vi "HSE Logger - Log Handlers and Levels.vi"(8 "error in":errorcluster) -> (0 "error out":errorcluster)   [LabVIEW 2024]
uses:
  <vilib>/Utility/error.llb/Trim Whitespace One-Sided.vi
  <vilib>/Hampel Software Engineering/HSE Logger/Handler/Handler.lvclass
  <vilib>/Hampel Software Engineering/HSE Logger/hse-logger.lvlib
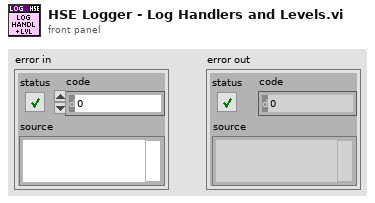
[diagram p1: front panel]
types:
  T1 = typedef "hse-logger.lvlib/LogLevel.ctl" = enum16{"DEBUG", "INFO", "WARNING", "ERROR", "CRITICAL"}
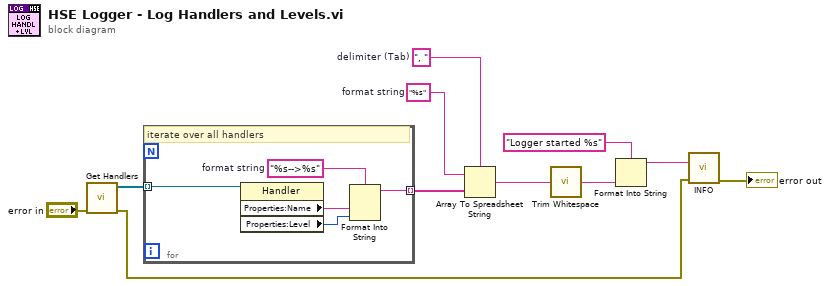
[diagram p0: block diagram]
diagram:
  w5 = ", "  # delimiter (Tab)
  w6 = "%s"  # format string
  n1 = call <vilib>:"Get Handlers.vi"("error in"="error in") -> ("error out"=w10:errorcluster, "Handlers"=w8:refnum<class "Handler.lvclass">[])  [unwired: 9 in]
  n2 = for {
    tunnel: w8 -> [w16] mode=indexing
    tunnel: [w12] -> w7 mode=indexing
    w15 = "%s-->%s"  # format string
    # "iterate over all handlers"
    n3 = property class="Handler"(reference=w16) -> ("Properties:Name"=w14:string, "Properties:Level"=w13:T1)  [unwired: 1 in, 2 out]
    n4 = Format Into String(format string=w15, w14, w13) -> (resulting string=w12:string)  [unwired: 2 in, 1 out]
  }
  n5 = Array To Spreadsheet String(delimiter (Tab)=w5, array=w7, 3:w6) -> (spreadsheet string=w4:string)
  n6 = call <vilib>:"Trim Whitespace.vi"("string"=w4) -> ("trimmed string"=w2:string)  [unwired: 1 in]
  n7 = Format Into String(format string="Logger started %s", w2) -> (resulting string=w1:string)  [unwired: 2 in, 1 out]
  n8 = call <vilib>:"INFO.vi"("Message"=w1, "error in"=w10) -> ("error out"=→"error out":errorcluster)  [unwired: 9 in]
